vi "Read Environment.vi"(8 "error in (no error)":errorcluster, 11 "WebView2 Control in":refnum<class "WebView2 Control.lvclass">) -> (0 "error out":errorcluster, 2 "Environment":refnum<k24>, 3 "WebView2 Control out":refnum<class "WebView2 Control.lvclass">)   [LabVIEW 2020, in "WebView2.lvlib" / "WebView2 Control.lvclass"]
uses:
  WebView2 Control.lvclass
  WebView2 Control.lvclass/WebView2 Control.ctl
  C:/Users/Simon/Documents/GitHub/LV-WebView2/Source/Libs/Microsoft.Web.WebView2.Core.dll
  Libs/Microsoft.Web.WebView2.Core.dll
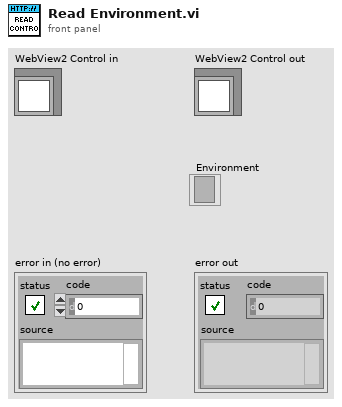
[diagram p1: front panel]
types:
  T1 = typedef "WebView2.lvlib/WebView2 Control.lvclass/Res.ctl" = cluster{"WebView2":refnum<k24>, "Webview2 Core":refnum<k24>, "event callback":refnum<k27>, "Environment":refnum<k24>}
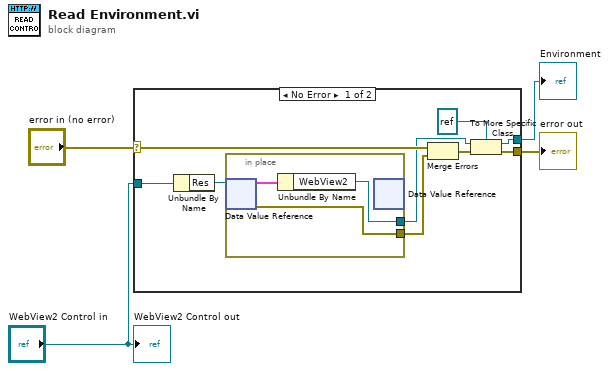
[diagram p0: block diagram]
diagram:
  n1 = case shown="No Error" "error in (no error)" {
    selector: "error in (no error)" -> [w13 w17]
    tunnel: [w6 _] -> w1
    tunnel: [w8 w17] -> w2
    tunnel: "WebView2 Control in" -> [w12 _]
    frame No Error {
      n2 = Unbundle By Name(w12) -> ("Res"=w11:refnum<data-value>)
      n3 = in-place {
        in-place-border: [w15] -> w7
        in-place-border: [w14] -> w9
        n4 = in-place-dvr #1(w11) -> (w16:T1, w14:errorcluster)
        n5 = Unbundle By Name(w16) -> ("WebView2"=w15:refnum<k24>)
        n6 = in-place-dvr #1() -> ()  [unwired: 1 in, 2 out]
      }
      n7 = Merge Errors(w13, w9) -> (w10:errorcluster)
      n8 = To More Specific Class(target class=refnum<k24> refnum ("Environment"), reference=w7, error in=w10) -> (specific class reference=w6:refnum<k24>, error out=w8:errorcluster)
    }
    frame Error {
    }
  }
  "error out" <- w2
  "Environment" <- w1
  "WebView2 Control out" <- "WebView2 Control in"
